vi "COMI Unload Device.vi"(11 "hDevice":u32) -> (3 "hDevice out":u32)   [LabVIEW 2017, in "Comidll.lvlib"]
doc: "void (COMI_UnloadDevice) (HANDLE hDevice);"
uses:
  <userlib>/Comidll/Comidll.lvlib
  <userlib>/Comidll/Comidll.dll
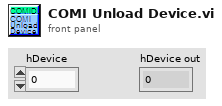
[diagram p1: front panel]
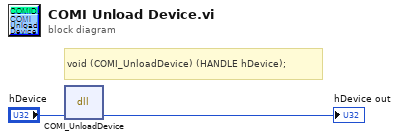
[diagram p0: block diagram]
diagram:
  # "void\t(COMI_UnloadDevice) (HANDLE hDevice);"
  n1 = dll-call lib="C:/Program Files/National Instruments/LabVIEW 2017/user.lib/Comidll/Comidll.*" fn="COMI_UnloadDevice"("hDevice"="hDevice") -> ("hDevice"=→"hDevice out":u32)  [unwired: 4 in, 2 out]
